vi "GPIO实验.vi"() -> ()   [LabVIEW 2011]
uses:
  <vilib>/eio/EIO_TerminalDirection.ctl
  <vilib>/STM32_DriverVI_Interface_F4/GPIO_EIO/GPO_EIO_Inner_F4.vi
  <vilib>/eio/EIONode/EIONode.xnode
  <vilib>/STM32_DriverVI_Interface_F4/GPIO/PortX_in_F4.ctl
  <vilib>/STM32_DriverVI_Interface_F4/GPIO/pin_in_F4.ctl
  <vilib>/STM32_DriverVI_Interface_F4/GPIO/GPO_Mode_Interface_F4.ctl
panel:
  in  "毫秒倍数 2":u32(slide) scale=200.0..2000.0
  in  "停止 2":bool
  out "数值 2":i32
  in  "毫秒倍数":u32(knob) scale=200.0..2000.0
  in  "停止":bool
  out "数值":i32
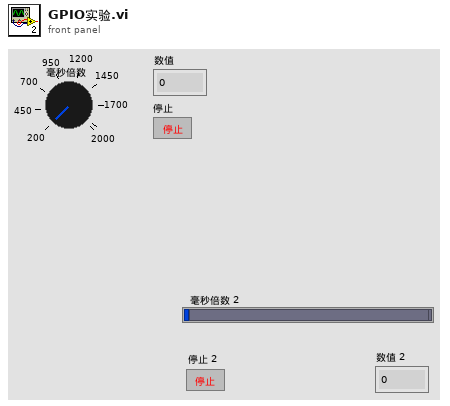
[diagram p1: front panel]
types:
  T1 = typedef "GPO_Mode_Interface_F4.ctl" = enum8{"Push-pull Output", "Open-drain Output"}
  T2 = typedef "pin_in_F4.ctl" = enum8{"P0", "P1", "P2", "P3", "P4", "P5", "P6", "P7", "P8", "P9", "P10", "P11", "P12", "P13", "P14", "P15"}
  T3 = typedef "PortX_in_F4.ctl" = enum8{"Port_A", "Port_B", "Port_C", "Port_D", "Port_E", "Port_F", "Port_G", "Port_H", "Port_I"}
  T4 = enum8{"P0", "P1", "P2", "P3", "P4", "P5", "P6", "P7", "P8", "P9", "P10", "P11", "P12", "P13", "P14", "P15"}
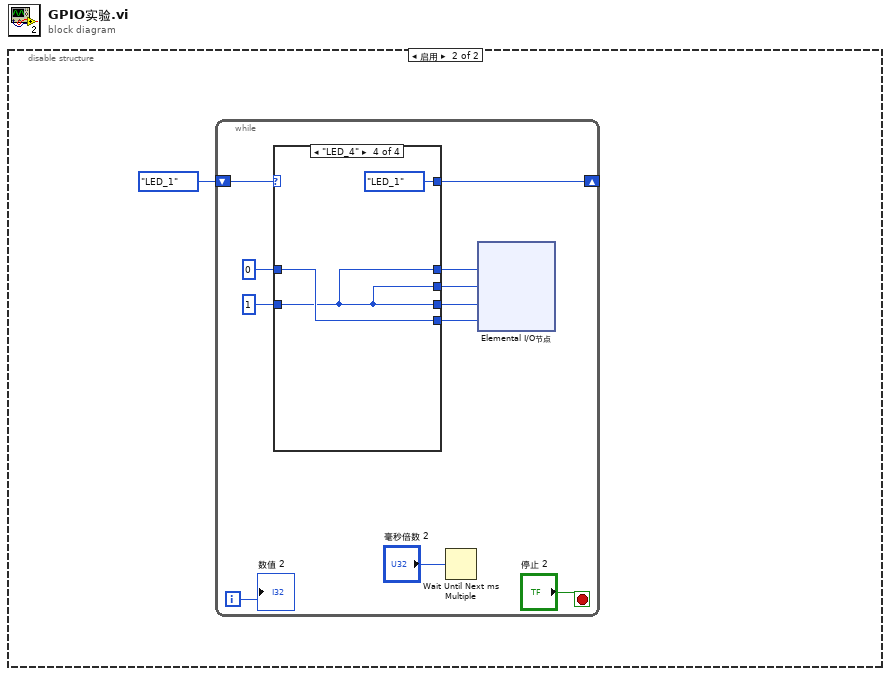
[diagram p0: block diagram]
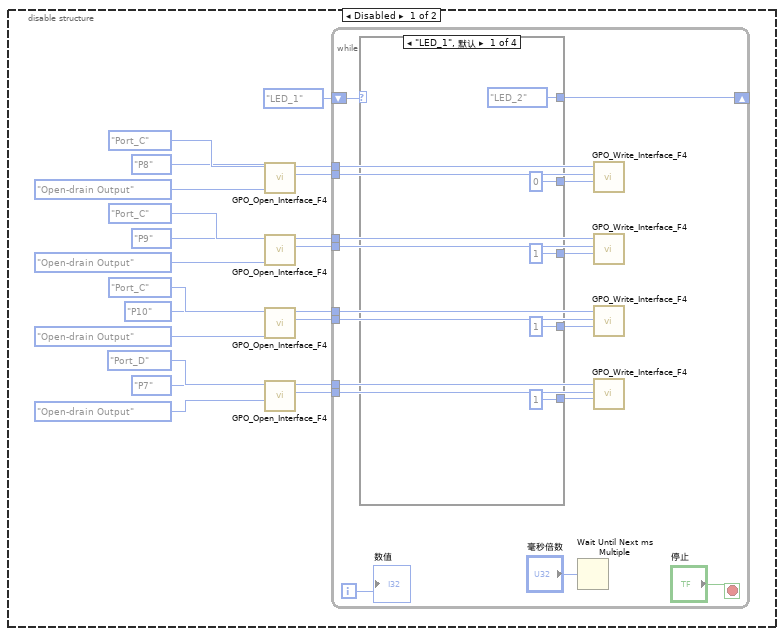
[diagram p2: hidden frame]
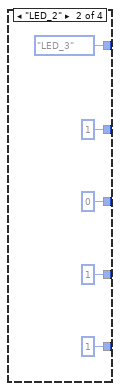
[diagram p3: hidden frame]
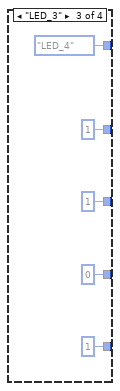
[diagram p4: hidden frame]
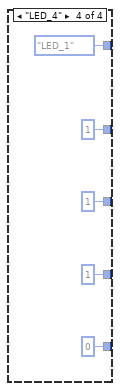
[diagram p5: hidden frame]
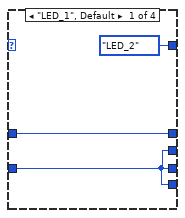
[diagram p6: hidden frame]
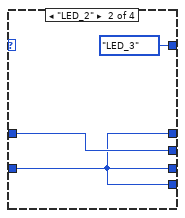
[diagram p7: hidden frame]
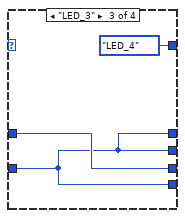
[diagram p8: hidden frame]
diagram:
  n1 = disable-structure shown="启用" {
    frame Disabled {
      n2 = call <vilib>:"GPO_Open_Interface_F4.vi"("mode"=GPO_Mode_Interface_F4."Open-drain Output", "pin_in"=pin_in_F4."P8", "PortX_in"=PortX_in_F4."Port_C") -> ("pin_out"=w7:u16, "PortX_out"=w8:u16)  [unwired: 6 in, 1 out]
      n3 = call <vilib>:"GPO_Open_Interface_F4.vi"("mode"=GPO_Mode_Interface_F4."Open-drain Output", "pin_in"=pin_in_F4."P9", "PortX_in"=PortX_in_F4."Port_C") -> ("pin_out"=w5:u16, "PortX_out"=w6:u16)  [unwired: 6 in, 1 out]
      n4 = call <vilib>:"GPO_Open_Interface_F4.vi"("mode"=GPO_Mode_Interface_F4."Open-drain Output", "pin_in"=pin_in_F4."P10", "PortX_in"=PortX_in_F4."Port_C") -> ("pin_out"=w3:u16, "PortX_out"=w4:u16)  [unwired: 6 in, 1 out]
      n5 = call <vilib>:"GPO_Open_Interface_F4.vi"("mode"=GPO_Mode_Interface_F4."Open-drain Output", "pin_in"=pin_in_F4."P7", "PortX_in"=PortX_in_F4."Port_D") -> ("pin_out"=w1:u16, "PortX_out"=w2:u16)  [unwired: 6 in, 1 out]
      n6 = while {
        tunnel: w8 -> [w33]
        tunnel: w7 -> [w32]
        tunnel: w6 -> [w31]
        tunnel: w5 -> [w30]
        tunnel: w4 -> [w28]
        tunnel: w3 -> [w29]
        tunnel: w2 -> [w35]
        tunnel: w1 -> [w34]
        shift-right: [w23] -> _
        shift-left: enum16{"LED_1", "LED_2", "LED_3", "LED_4"}."LED_1" -> [w36]
        i -> [w38]
        stop <- "停止" stop-if-true
        n7 = case shown="\"LED_1\", 默认" w36 {
          tunnel: [0 1 1 1] -> w27
          tunnel: [1 1 1 0] -> w26
          tunnel: [1 0 1 1] -> w25
          tunnel: [1 1 0 1] -> w24
          tunnel: [enum16{"LED_1", "LED_2", "LED_3", "LED_4"}."LED_2" enum16{"LED_1", "LED_2", "LED_3", "LED_4"}."LED_3" enum16{"LED_1", "LED_2", "LED_3", "LED_4"}."LED_4" enum16{"LED_1", "LED_2", "LED_3", "LED_4"}."LED_1"] -> w23
          frame "LED_1", Default {
          }
          frame "LED_2" {
          }
          frame "LED_3" {
          }
          frame "LED_4" {
          }
        }
        n8 = Wait Until Next ms Multiple(millisecond multiple="毫秒倍数") -> ()  [unwired: 1 out]
        n9 = call <vilib>:"GPO_Write_Interface_F4.vi"("Level_Value"=w27, "pin_in"=w32, "PortX_in"=w33) -> ()  [unwired: 6 in, 3 out]
        n10 = call <vilib>:"GPO_Write_Interface_F4.vi"("Level_Value"=w25, "pin_in"=w30, "PortX_in"=w31) -> ()  [unwired: 6 in, 3 out]
        n11 = call <vilib>:"GPO_Write_Interface_F4.vi"("Level_Value"=w24, "pin_in"=w29, "PortX_in"=w28) -> ()  [unwired: 6 in, 3 out]
        n12 = call <vilib>:"GPO_Write_Interface_F4.vi"("Level_Value"=w26, "pin_in"=w34, "PortX_in"=w35) -> ()  [unwired: 6 in, 3 out]
        "数值" <- w38
      }
    }
    frame Enabled {
      n13 = while {
        shift-right: [w69] -> _
        shift-left: enum16{"LED_1", "LED_2", "LED_3", "LED_4"}."LED_1" -> [w70]
        i -> [w62]
        stop <- "停止 2" stop-if-true
        n14 = case shown="\"LED_4\"" w70 {
          tunnel: [enum16{"LED_1", "LED_2", "LED_3", "LED_4"}."LED_2" enum16{"LED_1", "LED_2", "LED_3", "LED_4"}."LED_3" enum16{"LED_1", "LED_2", "LED_3", "LED_4"}."LED_4" enum16{"LED_1", "LED_2", "LED_3", "LED_4"}."LED_1"] -> w69
          tunnel: 0 -> [w88 w91 w94 w97]
          tunnel: 1 -> [w87 w90 w93 w96]
          tunnel: [w88 w90 w93 w96] -> w66
          tunnel: [w87 w90 w94 w96] -> w65
          tunnel: [w87 w90 w93 w97] -> w64
          tunnel: [w87 w91 w93 w96] -> w63
          frame "LED_1", Default {
          }
          frame "LED_2" {
          }
          frame "LED_3" {
          }
          frame "LED_4" {
          }
        }
        n15 = Wait Until Next ms Multiple(millisecond multiple="毫秒倍数 2") -> ()  [unwired: 1 out]
        n16 = xnode "Elemental I/O节点"("LED_1"=w66, "LED_2"=w63, "LED_3"=w65, "LED_4"=w64) -> ()  [unwired: 4 in, 4 out]
        "数值 2" <- w62
      }
    }
  }
